vi "Counter0.vi"() -> ()   [LabVIEW 2013]
uses:
  <vilib>/rvi/Emulation/niFpgaSctlEmulationGetInTimedLoop.vi
  <vilib>/rvi/Emulation/niFpgaEmulationReportErrorSimple.vi
  <vilib>/rvi/Emulation/niFpgaGetClockAttributes.vi
  <vilib>/rvi/eio/common/nirviEmuTemplateMethod_errors.vi
  <vilib>/rvi/Emulation/niFpgaCriticalErrorInLSC.vi
  <vilib>/eio/EIONode/EIONode.xnode
panel:
  out "Count Register":u8
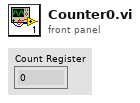
[diagram p1: front panel]
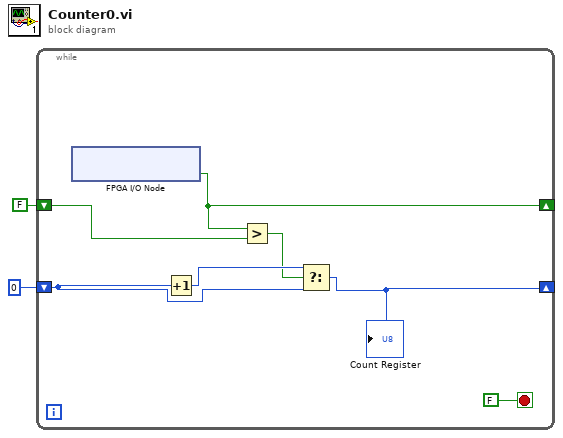
[diagram p0: block diagram]
diagram:
  n1 = while {
    shift-right: [w3] -> _
    shift-left: FALSE ("Connector0/DIO0") -> [w8]
    shift-right: [w4] -> _
    shift-left: u32 0 -> [w5]
    stop <- FALSE stop-if-true
    n2 = xnode "FPGA I/O Node"() -> ("Connector0/DIO0"=w3:bool)  [unwired: 1 in, 1 out]
    n3 = Increment(x=w5) -> (x+1=w7:u32)
    n4 = Greater?(x=w3, y=w8) -> (0:w6:bool)
    n5 = Select(t=w7, s=w6, f=w5) -> (s? t:f=w4:u32)
    "Count Register" <- w4
  }
